vi "Test Waveform Math.vi"() -> ()   [LabVIEW 2021]
uses:
  Source/Abs_Types/Waveform/Simple Read.vi
  Source/Constants/Support/WFM/Const_WFM.lvclass
  C:/TSA/LV_Abstract/Source/Abs_Types/Waveform/Abs_Waveform.lvclass
  Source/Constants/Support/WFM/WFM.vi
  Source/Functions/Math/Support/Add/WFM_Numeric/Method_Const.vi
  Source/Functions/Math/Support/Subtract/WFM_Numeric/Method_Const.vi
  Source/Abs_Types/Waveform/Abs_Waveform.lvclass
  <vilib>/measure/NI_MABase.lvlib
  Source/Functions/Math/Support/Add/WFM_Numeric/Add_WFM_Numeric.lvclass
  Source/Functions/Math/Support/Subtract/WFM_Numeric/Subtract_WFM_Numeric.lvclass
  C:/Program Files (x86)/National Instruments/LabVIEW 2021/vi.lib/TSA/Abstract Data Classes/Abs_Types/Value/Abs_Value.lvclass
  C:/Program Files (x86)/National Instruments/LabVIEW 2021/vi.lib/TSA/Abstract Data Classes/Abs_Types/Type/Abs_Type.lvclass
  C:/TSA/LV_Abstract/Source/Constants/Support/WFM/Const_WFM.lvclass
panel:
  out "Waveform Chart 2":waveform(dbl)(graph)
  out "Waveform Chart":waveform(dbl)(graph)
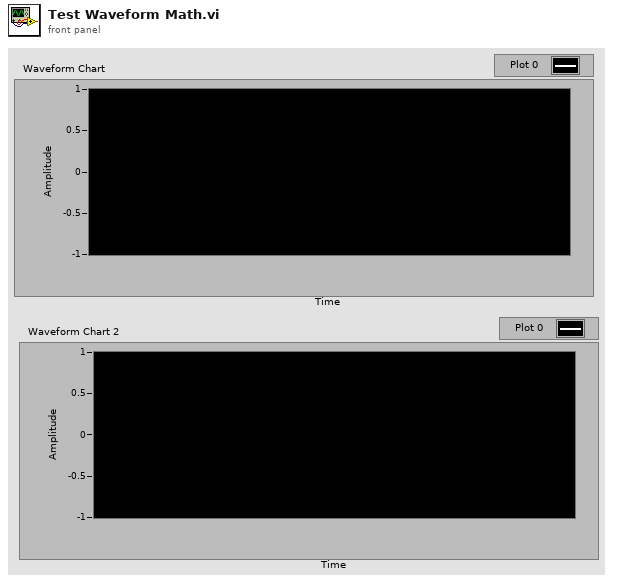
[diagram p1: front panel]
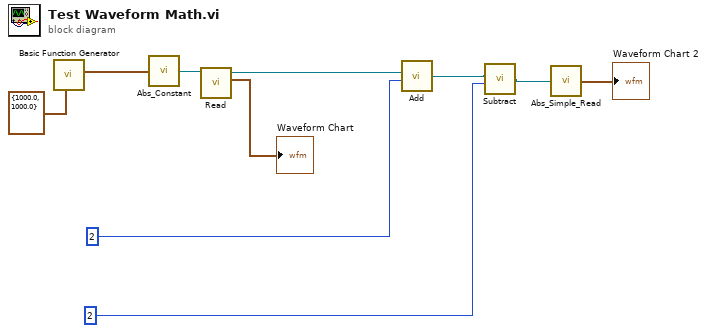
[diagram p0: block diagram]
diagram:
  n1 = call <vilib>:"Basic Function Generator.vi"("sampling info"=cluster{"Fs":dbl, "#s":dbl} {"Fs"=1000.0, "#s"=1000.0}) -> ("signal out"=w8:waveform(dbl))  [unwired: 8 in, 2 out]
  n2 = call-poly "Abs_Constant.vi"("Value"=w8) -> ("Constant"=w9:refnum<class "Const_WFM.lvclass">)  [unwired: 4 in]
  n3 = call-dynamic "Read.vi"("Const_WFM in"=w9) -> ("Waveform"=→"Waveform Chart":waveform(dbl), "Const_WFM out"=w6:refnum<class "Const_WFM.lvclass">)  [unwired: 8 in, 1 out]
  n4 = call-poly "Add.vi"("Value"=2, "Abs_Waveform.lvclass"=w6) -> ("Result"=w2:refnum<class "Abs_Waveform.lvclass">)  [unwired: 4 in]
  n5 = call-poly "Subtract.vi"("Value"=2, "Abs_Waveform.lvclass"=w2) -> ("Result"=w1:refnum<class "Abs_Waveform.lvclass">)  [unwired: 4 in]
  n6 = call-poly "Abs_Simple_Read.vi"("Abs_Waveform in"=w1) -> ("Waveform"=→"Waveform Chart 2":waveform(dbl))  [unwired: 4 in]
